vi "16IN16Out-Outbit.vi"(8 "error in (no error)":errorcluster, 10 "BL":bool, 11 "16InOut IO_Output":T1) -> (0 "error out":errorcluster)   [LabVIEW 2019]
uses:
  Ctrl/16InOut_SelectOutPut.ctl
  IO_Class/IOCard.lvclass
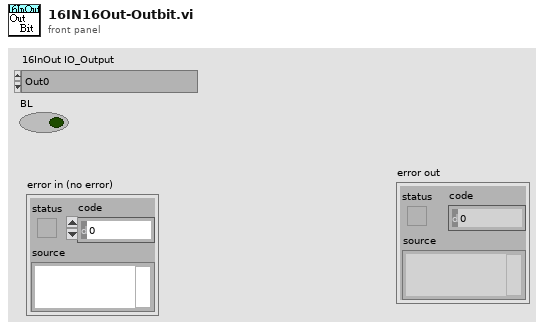
[diagram p1: front panel]
types:
  T1 = typedef "16InOut_SelectOutPut.ctl" = enum16{"Out0", "Out1", "Out2", "Out3", "Out4", "Out5", "Out6", "Out7", "Out8", "Out9", "Out10", "Out11", "Out12", "Out13", "Out14", "Out15"}
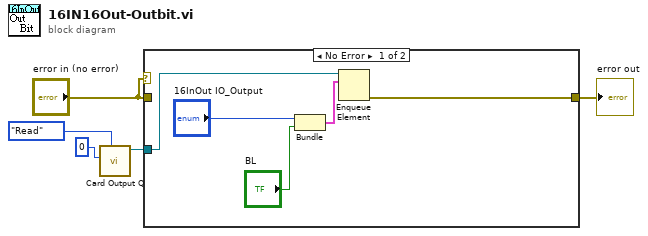
[diagram p0: block diagram]
diagram:
  n1 = call "Card Output Q.vi"("Action"=enum16{"Initial", "Write", "Read", "Release"}."Read", "CardIndex"=0) -> ("Output Q Out"=w1:refnum<queue>)  [unwired: 8 in, 1 out]
  n2 = case shown="No Error" "error in (no error)" {
    tunnel: "error in (no error)" -> [_ w11]
    tunnel: [w9 w11] -> w5
    tunnel: w1 -> [w10 _]
    frame No Error {
      n3 = Bundle("16InOut IO_Output"="16InOut IO_Output", "BL"="BL") -> (w6:cluster{"16InOut IO_Output":T1, "BL":bool})  [unwired: 1 in]
      n4 = Enqueue Element(queue=w10, element=w6) -> (error out=w9:errorcluster)  [unwired: 2 in, 2 out]
    }
    frame Error {
    }
  }
  "error out" <- w5
